vi "Psi (Digamma) Function.vi"(3 "x":dbl format="%.2f") -> (1 "y(x)":dbl format="%.2f")   [LabVIEW 2014, in "NI_Gmath.lvlib"]
doc: "Computes the psi, or digamma, function."
uses:
  NI_Gmath.lvlib
  lvanlys.dll
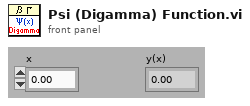
[diagram p1: front panel]
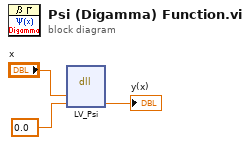
[diagram p0: block diagram]
diagram:
  n1 = dll-call lib="C:/Program Files (x86)/National Instruments/LabVIEW 2014/resource/lvanlys.*" fn="LV_Psi"("x"="x", "Psi(x)"=0.0 ("Psi")) -> ("Psi(x)"=→"y(x)":dbl)  [unwired: 5 in, 2 out]
